vi "Levitador.vi"() -> ()   [LabVIEW 2021]
uses:
  <vilib>/Instr/_visa.llb/VISA Configure Serial Port (Instr).vi
  <vilib>/addons/control/pid/pid.llb/PID (DBL).vi
  <vilib>/addons/control/pid/NI_PID_pid.lvlib
panel:
  out "Gráfica 2":dbl(graph)
  in  "y":dbl
  in  "x":dbl
  out "Salida 2":dbl
  out "Gráfica":cluster{dbl, dbl}(graph)
  out "Salida":dbl
  in  "stop":bool
  in  "PID gains":T1={"Kp"=1.0, "Ti"=0.01, "Td"=0.0, "Referencia"=0.0, "T Muestreo"=0.0} {"T Muestreo" scale=0.0..1000.0; "Referencia" scale=0.0..360.0; "Td" format="%.3f"; "Ti" format="%.3f"; "Kp" format="%.3f"}
  in  "VISA resource name":refnum<visa-resource-name>
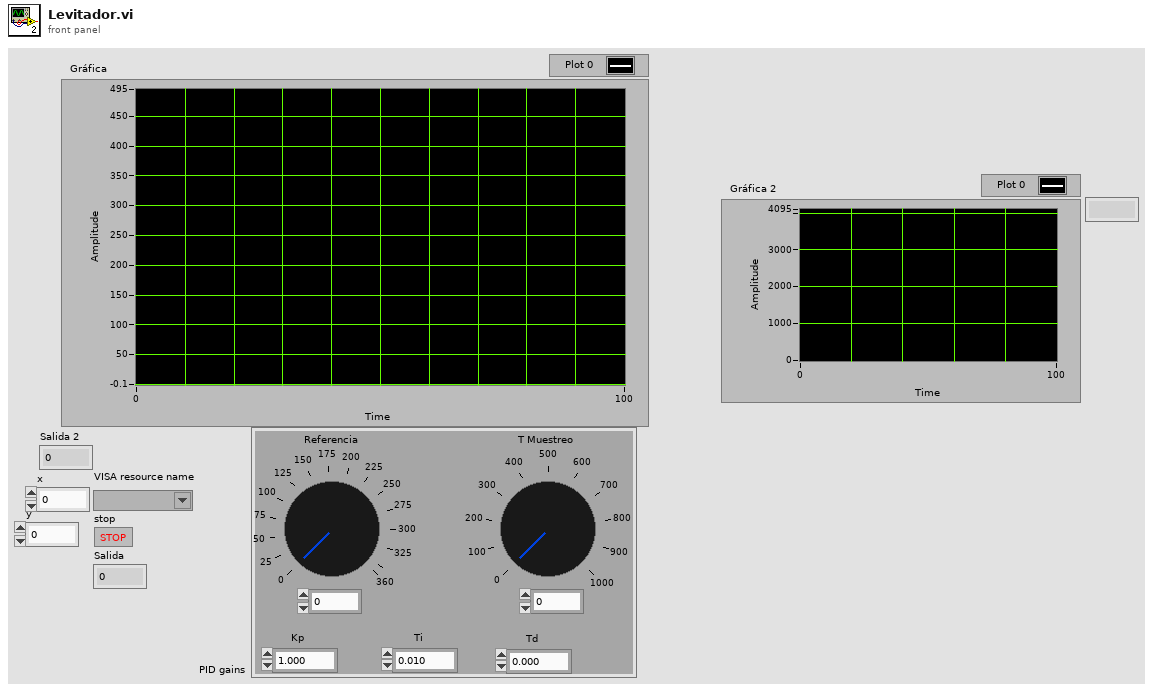
[diagram p1: front panel]
types:
  T1 = cluster{"Kp":dbl, "Ti":dbl, "Td":dbl, "Referencia":dbl, "T Muestreo":dbl}
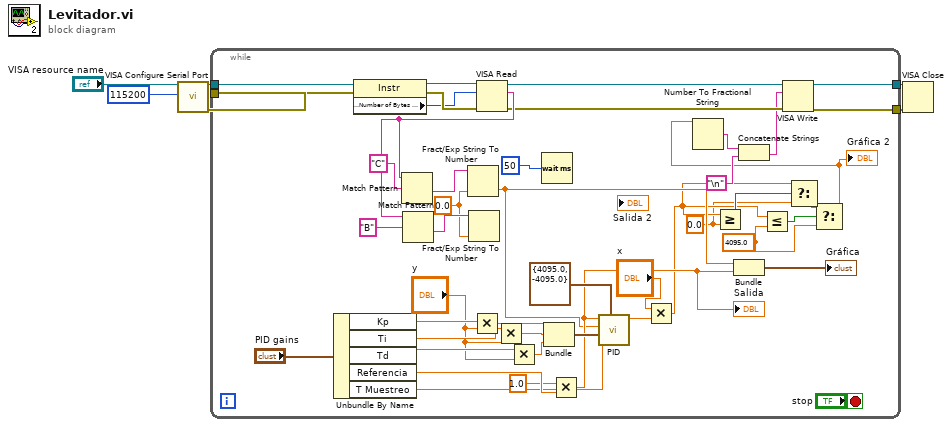
[diagram p0: block diagram]
diagram:
  n1 = call-poly "VISA Configure Serial Port"("VISA resource name"="VISA resource name", "baud rate (9600)"=u32 115200) -> ("VISA resource name out"=w4:refnum<visa-resource-name>, "error out"=w3:errorcluster)  [unwired: 12 in]
  n2 = while {
    tunnel: w4 -> [w51]
    tunnel: w3 -> [w50]
    tunnel: [w38] -> w2
    tunnel: [w37] -> w1
    stop <- "stop" stop-if-true
    w12 = 4095.0 ("y")
    w8 = 0.0 ("y")
    w41 = 0.0 ("default (0 DBL)")
    n3 = Unbundle By Name("PID gains") -> ("Kp"=w21:dbl, "Ti"=w19:dbl, "Td"=w18:dbl, "Referencia"=w33:dbl, "T Muestreo"=w7:dbl)
    n4 = property class="Instr"(reference=w51, error in=w50) -> (reference out=w49:refnum<visa-resource-name>, error out=w48:errorcluster, "Serial Settings:Number of Bytes at Serial Port"=w47:u32)
    n5 = Multiply(x=w21, y="y") -> (x*y=w20:dbl)
    n6 = VISA Read(VISA resource name=w49, byte count=w47, error in (no error)=w48) -> (VISA resource name out=w40:refnum<visa-resource-name>, read buffer=w46:string, error out=w39:errorcluster)  [unwired: 1 out]
    n7 = Match Pattern(string=w46, regular expression="C") -> (after substring=w43:string)  [unwired: 1 in, 3 out]
    n8 = Match Pattern(string=w46, regular expression="B") -> (after substring=w42:string)  [unwired: 1 in, 3 out]
    n9 = Fract/Exp String To Number(string=w43, default (0 dbl)=w41) -> (number=w24:dbl)  [unwired: 2 in, 1 out]
    n10 = Fract/Exp String To Number(string=w42, default (0 dbl)=w41) -> ()  [unwired: 2 in, 2 out]
    n11 = Multiply(x=w19, y="y") -> (x*y=w16:dbl)
    n12 = Multiply(x=w18, y="y") -> (x*y=w15:dbl)
    n13 = Wait (ms)(milliseconds to wait=u32 50) -> ()  [unwired: 1 out]
    n14 = Bundle(w20, w16, w15) -> (w34:cluster{dbl, dbl, dbl})  [unwired: 1 in]
    n15 = Multiply(x=1.0 ("y"), y=w33) -> (x*y=w30:dbl)
    "Salida" <- w30
    n16 = call-poly <vilib>:"PID.vi"("output range"=cluster{"output high":dbl, "output low":dbl} {"output high"=4095.0, "output low"=-4095.0}, "dt (s)"=w7, "PID gains"=w34, "process variable"=w24, "setpoint"=w30) -> ("output"=w31:dbl)  [unwired: 5 in, 1 out]
    n17 = Multiply(x="x", y=w31) -> (x*y=w9:dbl)
    n18 = Greater Or Equal?(x=w9, y=w8) -> (x >= y?=w14:bool)
    n19 = Bundle(w24, w30) -> (→"Gráfica":cluster{dbl, dbl})  [unwired: 1 in]
    n20 = Less Or Equal?(x=w9, y=w12) -> (x <= y?=w13:bool)
    n21 = Select(t=w9, s=w14, f=w8) -> (s? t:f=w11:dbl)
    n22 = Select(t=w11, s=w13, f=w12) -> (s? t:f=w10:dbl)
    "Gráfica 2" <- w10
    n23 = Number To Fractional String(number=w10) -> (F-format string=w27:string)  [unwired: 3 in]
    n24 = Concatenate Strings(w27, "\n") -> (w25:string)
    n25 = VISA Write(VISA resource name=w40, write buffer=w25, error in (no error)=w39) -> (VISA resource name out=w38:refnum<visa-resource-name>, error out=w37:errorcluster)  [unwired: 1 out]
  }
  n26 = VISA Close(VISA resource name=w2, error in (no error)=w1) -> ()  [unwired: 1 out]
